vi "Replace Characters - backup.vi"(0 "String In":string) -> (2 "String Out":string)   [LabVIEW 2020]
doc: "This VI was created for use with the Read/Write Cluster VIs. It converts any carriage returns and line feeds in the string to unique identifier strings which can be converted back upon reading the file.\n\nFreeware from Moore Good Ideas, www.mooregoodideas.com. Do not remove this line."
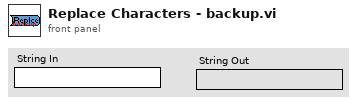
[diagram p1: front panel]
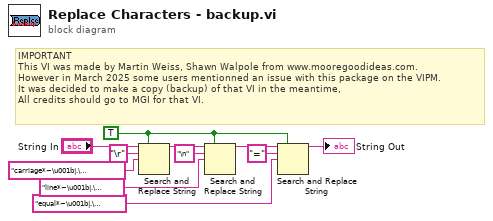
[diagram p0: block diagram]
diagram:
  w3 = TRUE ("replace all? (F)")
  # "IMPORTANT\nThis VI was made by Martin Weiss, Shawn Walpole from www.mooregoodideas.com.\nHowever in March 2025 some users mentionned an issue with this package on the VIPM.\nIt was decided to make a copy (backup) of that VI in the meantime,\nAll credits should go to MGI for that VI."
  n1 = Search and Replace String(replace all?=w3, input string="String In", search string="\r" ("replace string (\"\")"), replace string="carriage*~\u001b|.\u0017return") -> (result string=w8:string)  [unwired: 4 in, 3 out]
  n2 = Search and Replace String(replace all?=w3, input string=w8, search string="\n" ("replace string (\"\")"), replace string="line*~\u001b|.\u0017feed") -> (result string=w4:string)  [unwired: 4 in, 3 out]
  n3 = Search and Replace String(replace all?=w3, input string=w4, search string="=" ("replace string (\"\")"), replace string="equal*~\u001b|.\u0017sign") -> (result string=→"String Out":string)  [unwired: 4 in, 3 out]
